vi "OnshapeAngles.vi"   [LabVIEW 2020]
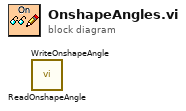
[diagram p0: block diagram]
diagram:
  n1 = call "ReadOnshapeAngle.vi"() -> ()  [unwired: 9 in, 3 out]
  n2 = call "WriteOnshapeAngle.vi"() -> ()  [unwired: 11 in, 1 out]
